vi "Add Buffers with Children.vi"(1 "byte order":T1, 4 "channels":T2[](array[typedef]) {"string offset" format="%d bytes"}, 5 "inline":bool, 6 "Decimation":u64, 7 "Transfer Group Status":refnum<class "Status.lvclass">, 8 "error in (no error)":errorcluster, 9 "Buffers":refnum<class "Buffers.lvclass">, 10 "parent tag":string, 11 "Application Data In":T5) -> (0 "error out":errorcluster, 3 "Application Data out":T5)   [LabVIEW 2017, in "DSF Core.lvlib"]
uses:
  DSF Core.lvlib
  Main VI/Application Data.ctl
  <vilib>/NI/Memory Manager/Classes/Pointer/Pointer.lvclass
  Classes/Framework/Framework.lvclass
  Buffer Reader/Buffer Data.ctl
  Classes/Buffer/Buffer.lvclass
  C:/Program Files (x86)/National Instruments/LabVIEW 2017/vi.lib/NI/Memory Manager/Classes/Pointer/Pointer.lvclass
  Classes/Transfer Group Status/Status.lvclass
  Typedefs/DSF Data Type.ctl
  Typedefs/DSF Engine Channel Configuration.ctl
  Typedefs/DSF Settings Info.ctl
  Typedefs/DSF Byte Order.ctl
  Typedefs/DSF Engine Framework Configuration.ctl
  Typedefs/DSF Engine Plugin Configuration.ctl
  Typedefs/DSF Timing Info.ctl
  Typedefs/DSF Engine Plugin Thread Configuration.ctl
  Typedefs/DSF Engine Transfer Group Configuration.ctl
  Typedefs/DSF Direction.ctl
  Typedefs/DSF Engine Transfer Configuration.ctl
  Typedefs/DSF Timeout Behavior.ctl
  Classes/Buffers/Buffers.lvclass
  ID to Tree Items/Tree Item Type.ctl
  Classes/Buffers/Buffers.lvclass/Buffers.ctl
  <vilib>/NI/Memory Manager/Classes/Pointer/Pointer.lvclass/Pointer.ctl
  Classes/Buffer/Get Buffer Size.vi
  Sizeof.vi
  <vilib>/NI/Memory Manager/Classes/Pointer/Get Size.vi
  Classes/Buffer/Subset Buffer.vi
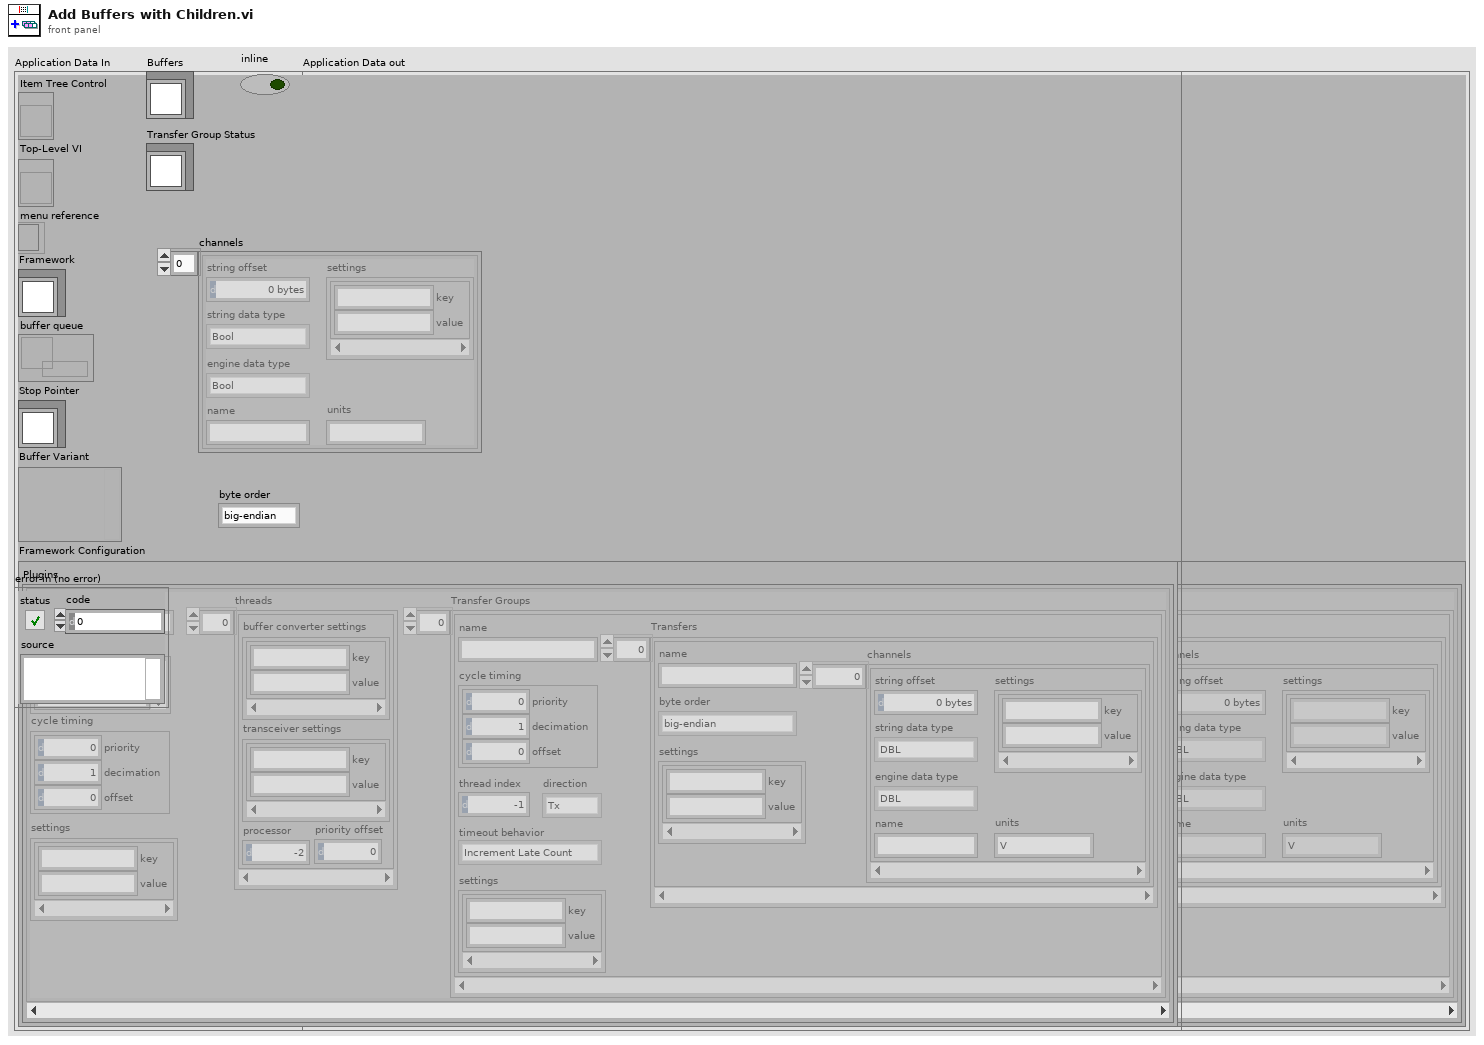
[diagram p1: front panel]
types:
  T1 = typedef "DSF Core.lvlib/DSF Byte Order.ctl" = enum8{"big-endian", "little-endian"}
  T2 = typedef "DSF Core.lvlib/DSF Engine Channel Configuration.ctl" = cluster{"string offset":u64, "string data type":T3, "engine data type":T3, "name":string, "settings":T4, "units":string}
  T3 = typedef "DSF Core.lvlib/DSF Data Type.ctl" = enum8{"Bool", "SGL", "DBL", "I8", "I16", "I32", "I64", "U8", "U16", "U32", "U64"}
  T4 = typedef "DSF Core.lvlib/DSF Settings Info.ctl" = cluster{"key":string, "value":string}[]
  T5 = typedef "DSF Core.lvlib/Application Data.ctl" = cluster{"Item Tree Control":refnum<vi>, "Top-Level VI":refnum<vi>, "menu reference":refnum<k9>, "Framework":refnum<class "Framework.lvclass">, "buffer queue":refnum<queue>, "Stop Pointer":refnum<class "Pointer.lvclass">, "Buffer Variant":variant, "Framework Configuration":T6}
  T6 = typedef "DSF Core.lvlib/DSF Engine Framework Configuration.ctl" = cluster{"Plugins":T7[]}
  T7 = typedef "DSF Core.lvlib/DSF Engine Plugin Configuration.ctl" = cluster{"name":string, "components":string[], "cycle timing":T8, "threads":T9[], "Transfer Groups":T10[], "settings":T4}
  T8 = typedef "DSF Core.lvlib/DSF Timing Info.ctl" = cluster{"priority":u64, "decimation":u64, "offset":u64}
  T9 = typedef "DSF Core.lvlib/DSF Engine Plugin Thread Configuration.ctl" = cluster{"buffer converter settings":T4, "transceiver settings":T4, "processor":i32, "priority offset":i16}
  T10 = typedef "DSF Core.lvlib/DSF Engine Transfer Group Configuration.ctl" = cluster{"name":string, "direction":T11, "cycle timing":T8, "thread index":i32, "settings":T4, "Transfers":T12[], "timeout behavior":T13}
  T11 = typedef "DSF Core.lvlib/DSF Direction.ctl" = enum8{"Tx", "Rx"}
  T12 = typedef "DSF Core.lvlib/DSF Engine Transfer Configuration.ctl" = cluster{"name":string, "byte order":T1, "settings":T4, "channels":T2[]}
  T13 = typedef "DSF Core.lvlib/DSF Timeout Behavior.ctl" = enum8{"Increment Late Count", "Throw Error"}
  T14 = typedef "DSF Core.lvlib/Buffer Data.ctl" = cluster{"Buffer":refnum<class "Buffer.lvclass">, "Status":refnum<class "Status.lvclass">, "decimation":u64, "avg bandwidth":dbl, "data type":T3, "units":string, "channels":T2[], "channel":bool, "engine (T) / string (F)":bool, "byte order":T1}
  T15 = typedef "DSF Core.lvlib/Tree Item Type.ctl" = enum16{"Framework", "Plugin Group", "Plugin", "Group", "Transfer", "Buffer", "Channel"}
  T16 = typedef "DSF Core.lvlib/Tree Item.ctl" = cluster{"Left Cell String":string, "Child Text":string[], "Child Tag":string, "Glyph Index":i32}
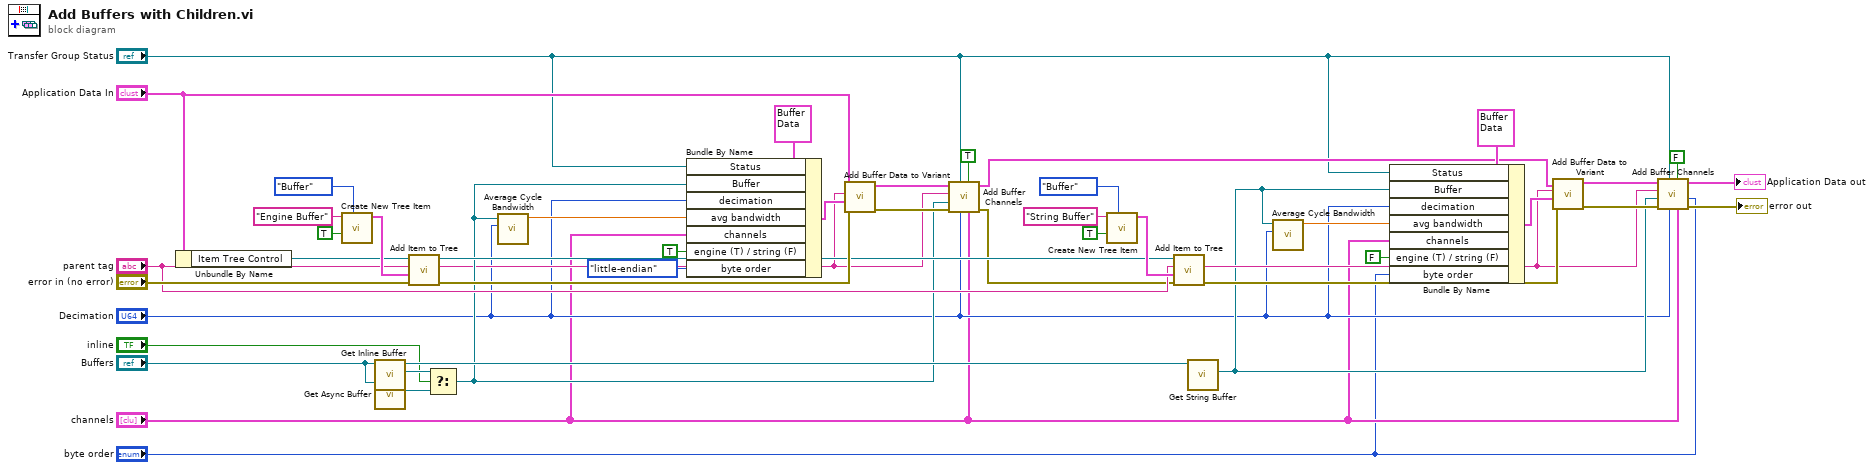
[diagram p0: block diagram]
diagram:
  n1 = Unbundle By Name("Application Data In") -> ("Item Tree Control"=w29:refnum<vi>)
  n2 = call "Create New Tree Item.vi"("Item Type"=Tree_Item_Type."Buffer", "found?"=TRUE, "Left Cell String"="Engine Buffer") -> ("Item"=w31:T16)  [unwired: 7 in, 1 out]
  n3 = call "Get Inline Buffer.vi"("Buffers in"="Buffers") -> ("Inline Buffer"=w23:refnum<class "Buffer.lvclass">, "Buffers out"=w38:refnum<class "Buffers.lvclass">)  [unwired: 9 in]
  n4 = call "Get Async Buffer.vi"("Buffers in"="Buffers") -> ("Async Buffer"=w24:refnum<class "Buffer.lvclass">)  [unwired: 9 in, 1 out]
  n5 = call "Add Item to Tree.vi"("error in (no error)"="error in (no error)", "Item"=w31, "parent tag"="parent tag", "TreeControl in"=w29) -> ("error out"=w44:errorcluster, "new item tag"=w16:string, "TreeControl out"=w39:refnum<vi>)  [unwired: 5 in]
  n6 = Select(t=w23, s="inline", f=w24) -> (s? t:f=w17:refnum<class "Buffer.lvclass">)
  n7 = call "Average Cycle Bandwidth.vi"("Decimation"="Decimation", "Buffer"=w17) -> ("avergage cycle bandwidth"=w27:dbl)  [unwired: 9 in]
  n8 = Bundle By Name(cluster=T14 {"Buffer"=refnum, "Status"=refnum, "decimation"=0, "avg bandwidth"=0.0, "data type"=enum."Bool", "units"="", "channels"=[], "channel"=FALSE, "engine (T) / string (F)"=FALSE, "byte order"=enum."little-endian"} ("Buffer data"), "Status"="Transfer Group Status", "Buffer"=w17, "decimation"="Decimation", "avg bandwidth"=w27, "channels"="channels", "engine (T) / string (F)"=TRUE, "byte order"=DSF_Byte_Order."little-endian") -> (w43:T14)
  n9 = call "Add Buffer Data to Variant.vi"("error in (no error)"=w44, "Buffer data"=w43, "tag"=w16, "Application Data In in"="Application Data In") -> ("error out"=w19:errorcluster, "Application Data In out"=w21:T5)  [unwired: 6 in]
  n10 = call "Add Buffer Channels.vi"("channels"="channels", "engine (T) / string (F)"=TRUE, "Decimation"="Decimation", "Transfer Group Status"="Transfer Group Status", "error in (no error)"=w19, "Buffer"=w17, "parent tag"=w16, "Application Data In"=w21) -> ("error out"=w18:errorcluster, "Application Data out"=w20:T5)  [unwired: 2 in]
  n11 = call "Create New Tree Item.vi"("Item Type"=Tree_Item_Type."Buffer", "found?"=TRUE, "Left Cell String"="String Buffer") -> ("Item"=w40:T16)  [unwired: 7 in, 1 out]
  n12 = call "Add Item to Tree.vi"("error in (no error)"=w18, "Item"=w40, "parent tag"="parent tag", "TreeControl in"=w39) -> ("error out"=w47:errorcluster, "new item tag"=w10:string)  [unwired: 5 in, 1 out]
  n13 = call "Get String Buffer.vi"("Buffers in"=w38) -> ("String Buffer"=w9:refnum<class "Buffer.lvclass">)  [unwired: 9 in, 1 out]
  n14 = call "Average Cycle Bandwidth.vi"("Decimation"="Decimation", "Buffer"=w9) -> ("avergage cycle bandwidth"=w26:dbl)  [unwired: 9 in]
  n15 = Bundle By Name(cluster=T14 {"Buffer"=refnum, "Status"=refnum, "decimation"=0, "avg bandwidth"=0.0, "data type"=enum."Bool", "units"="", "channels"=[], "channel"=FALSE, "engine (T) / string (F)"=FALSE, "byte order"=enum."little-endian"} ("Buffer data"), "Status"="Transfer Group Status", "Buffer"=w9, "decimation"="Decimation", "avg bandwidth"=w26, "channels"="channels", "engine (T) / string (F)"=FALSE, "byte order"="byte order") -> (w46:T14)
  n16 = call "Add Buffer Data to Variant.vi"("error in (no error)"=w47, "Buffer data"=w46, "tag"=w10, "Application Data In in"=w20) -> ("error out"=w12:errorcluster, "Application Data In out"=w14:T5)  [unwired: 6 in]
  n17 = call "Add Buffer Channels.vi"("byte order"="byte order", "channels"="channels", "engine (T) / string (F)"=FALSE, "Decimation"="Decimation", "Transfer Group Status"="Transfer Group Status", "error in (no error)"=w12, "Buffer"=w9, "parent tag"=w10, "Application Data In"=w14) -> ("error out"=→"error out":errorcluster, "Application Data out"=→"Application Data out":T5)  [unwired: 1 in]
